vi "Get Current Time.vi"() -> (6 "Time String":string)   [LabVIEW 2022 SP3]
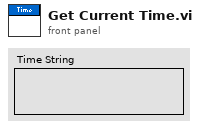
[diagram p1: front panel]
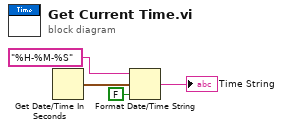
[diagram p0: block diagram]
diagram:
  n1 = Get Date/Time In Seconds() -> (seconds since 1Jan1904=w1:timestamp)
  n2 = Format Date/Time String(time format string (%c)="%H-%M-%S", seconds (now)=w1, UTC format=FALSE) -> (date/time string=→"Time String":string)
